vi "I2C_read_SubVI.vi"(9 "min time SCL Low (uSEC)":u32, 10 "min time SCL High (uSEC)":u32, 11 "number of bytes":i16) -> (3 "Data bit array":bool[](array[boolean]))   [LabVIEW 2019]
uses:
  <vilib>/rvi/Emulation/niFpgaGetClockAttributes.vi
  <vilib>/rvi/Emulation/niFpgaSctlEmulationGetInTimedLoop.vi
  <vilib>/rvi/Emulation/niFpgaEmulationReportErrorSimple.vi
  <vilib>/rvi/eio/common/nirviEmuTemplateMethod_errors.vi
  <vilib>/rvi/Emulation/niFpgaCriticalErrorInLSC.vi
  <vilib>/eio/EIONode/EIONode.xnode
panel:
  out "is last byte ?":bool
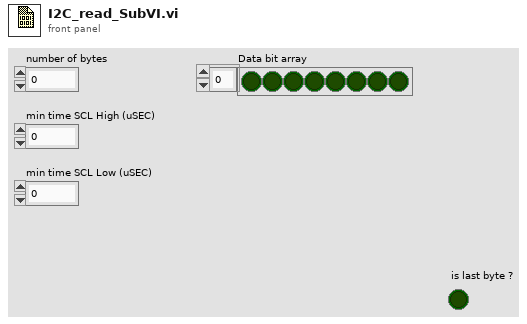
[diagram p1: front panel]
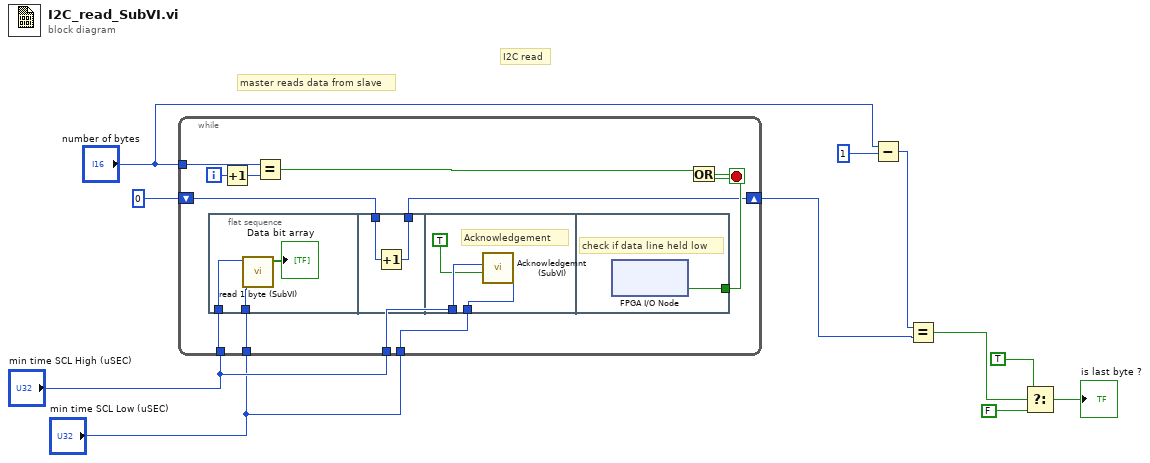
[diagram p0: block diagram]
diagram:
  # "I2C read"
  # "master reads data from slave"
  n1 = while {
    tunnel: "number of bytes" -> [w23]
    tunnel: "min time SCL High (uSEC)" -> [w17]
    tunnel: "min time SCL Low (uSEC)" -> [w16]
    tunnel: "min time SCL Low (uSEC)" -> [w15]
    tunnel: "min time SCL High (uSEC)" -> [w14]
    shift-right: [w13] -> w8
    shift-left: i16 0 -> [w12]
    i -> [w22]
    stop <- w19 stop-if-true
    n2 = flat-sequence {
      tunnel: w17 -> [w26]
      tunnel: w16 -> [w25]
      tunnel: [w28] -> w13
      tunnel: w12 -> [w27]
      tunnel: w15 -> [w31]
      tunnel: w14 -> [w30]
      tunnel: [w32] -> w18
      frame #0 {
        n3 = call "read 1 byte (SubVI).vi"("min time SCL Low (uSEC)"=w25, "min time SCL High (uSEC)"=w26) -> ("Data bit array"=→"Data bit array":bool[])  [unwired: 9 in]
      }
      frame #1 {
        n4 = Increment(x=w27) -> (x+1=w28:i16)
      }
      frame #2 {
        # "Acknowledgement"
        n5 = call "Acknowledgemnt (SubVI).vi"("Acknowledgement"=TRUE, "min time SCL High (uSEC)"=w30, "min time SCL Low (uSEC)"=w31) -> ()  [unwired: 9 in]
      }
      frame #3 {
        # "check if data line held low"
        n6 = xnode "FPGA I/O Node"() -> ("SDA"=w32:bool)  [unwired: 1 in, 1 out]
      }
    }
    n7 = Increment(x=w22) -> (x+1=w21:i32)
    n8 = Equal?(x=w23, y=w21) -> (x = y?=w20:bool)
    n9 = Or(x=w20, y=w18) -> (x .or. y?=w19:bool)
  }
  n10 = Subtract(x="number of bytes", y=i16 1) -> (x-y=w6:i16)
  n11 = Equal?(x=w6, y=w8) -> (x = y?=w2:bool)
  n12 = Select(t=TRUE, s=w2, f=FALSE) -> (s? t:f=→"is last byte ?":bool)
